vi "Create.vi"(5 "Name":string, 9 "Center":cluster{"x":i16, "y":i16}) -> (4 "FSM.Node":refnum<class "FSM.Node.lvclass">)   [LabVIEW 2020, in "FSM.Node.lvclass"]
uses:
  FSM.Node.lvclass
  Shape.ctl
  FSM.Node.lvclass/FSM.Node.ctl
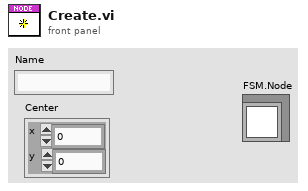
[diagram p1: front panel]
types:
  T1 = typedef "FSM.Node.lvclass/Shape.ctl" = enum16{"Default", "Start", "Action", "End"}
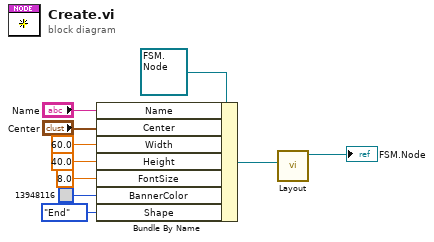
[diagram p0: block diagram]
diagram:
  n1 = Bundle By Name(cluster=refnum<class "FSM.Node.lvclass"> refnum ("FSM.Node"), "Name"="Name", "Center"="Center", "Width"=60.0 ("Serialized.Width"), "Height"=40.0 ("Serialized.Height"), "FontSize"=8.0 ("Serialized.FontSize"), "BannerColor"=u32 13948116, "Shape"=Shape."End" ("Serialized.Shape")) -> (w3:refnum<class "FSM.Node.lvclass">)
  n2 = call "Layout.vi"("FSM in"=w3) -> ("FSM out"=→"FSM.Node":refnum<class "FSM.Node.lvclass">)  [unwired: 9 in, 1 out]
